vi "Get Level.vi"(6 "Output Channel":T1, 8 "error in (no error)":errorcluster, 11 "Inst.RP100 in":refnum<class "Inst.RP100.lvclass">) -> (0 "error out":errorcluster, 2 "Level (V)":dbl, 3 "Inst.RP100 out":refnum<class "Inst.RP100.lvclass">)   [LabVIEW 2019, in "Inst.RP100.lvclass"]
uses:
  Inst.RP100.lvclass
  C:/Program Files (x86)/National Instruments/LabVIEW 2019/user.lib/LevyLab/Instrument Framework/SMOs/Instrument/Instrument.lvclass
  Typedefs/Output Channel--Enum.ctl
  Typedefs/Commands--Enum.ctl
  Typedefs/getLevel--Cluster.ctl
  <userlib>/LevyLab/Instrument Framework/SMOs/Instrument/Instrument.lvclass/Instrument.ctl
  01165c8c-b2e8-49b8-96e8-536698999359.vi/012e8175-f6b3-4063-807e-eae00dfba7fe.vi
  01165c8c-b2e8-49b8-96e8-536698999359.vi/012e8175-f6b3-4063-807e-eae00dfba7fe.vi/41478f01-57f4-4188-8f0a-c43f95c8f48e.vi
  <userlib>/LevyLab/Instrument Framework/SMOs/Instrument/API/Send and Receive.vi
  01165c8c-b2e8-49b8-96e8-536698999359.vi/012e8175-f6b3-4063-807e-eae00dfba7fe.vi/390a0fe6-66d0-4b1f-8944-62df44ed410c.vi
  <userlib>/LevyLab/Instrument Framework/SMOs/Instrument/Private/Get Client Type.vi
  01165c8c-b2e8-49b8-96e8-536698999359.vi/012e8175-f6b3-4063-807e-eae00dfba7fe.vi/41478f01-57f4-4188-8f0a-c43f95c8f48e.vi/d4522e91-9053-4c0e-9d1f-c7c48f8b6bcc.vi
  01165c8c-b2e8-49b8-96e8-536698999359.vi/012e8175-f6b3-4063-807e-eae00dfba7fe.vi/41478f01-57f4-4188-8f0a-c43f95c8f48e.vi/891fa407-0db4-4b04-91cd-89da5eed44a8.vi
  01165c8c-b2e8-49b8-96e8-536698999359.vi/012e8175-f6b3-4063-807e-eae00dfba7fe.vi/390a0fe6-66d0-4b1f-8944-62df44ed410c.vi/4d54c90f-f017-4dd3-9061-6dca01a9e2e0.vi
  01165c8c-b2e8-49b8-96e8-536698999359.vi/012e8175-f6b3-4063-807e-eae00dfba7fe.vi/390a0fe6-66d0-4b1f-8944-62df44ed410c.vi/c432f00d-fbcb-44ec-80e1-5223097179db.vi
  01165c8c-b2e8-49b8-96e8-536698999359.vi/012e8175-f6b3-4063-807e-eae00dfba7fe.vi/390a0fe6-66d0-4b1f-8944-62df44ed410c.vi/4d54c90f-f017-4dd3-9061-6dca01a9e2e0.vi/4a32ab2b-883d-45ba-8bf7-73b0a157e865.vi
  01165c8c-b2e8-49b8-96e8-536698999359.vi/012e8175-f6b3-4063-807e-eae00dfba7fe.vi/390a0fe6-66d0-4b1f-8944-62df44ed410c.vi/4d54c90f-f017-4dd3-9061-6dca01a9e2e0.vi/9b068e5f-e603-4ccd-b66b-d4bd0b9420a9.vi
  <userlib>/LevyLab/Instrument Framework/SMOs/Instrument/Private/Get RC Connection Status.vi
  <userlib>/LevyLab/Instrument Framework/SMOs/Instrument/API/Enum to String.vi
  <userlib>/LevyLab/Instrument Framework/SMOs/RemoteControl/API/Send and Receive.vi
  <vilib>/Utility/Data Type/Get Type Information.vi
  <vilib>/JDP Science/JSONtext/JSON text to Variant.vi
  <userlib>/LevyLab/Instrument Framework/SMOs/Instrument/API/Instrument.GetPublicEvents.vi
  <vilib>/JDP Science/JSONtext/Variant to JSON Text.vi
  <vilib>/National Instruments/GUID Generator/Guid Generator.vi
  <userlib>/LevyLab/Instrument Framework/SMOs/Instrument/API/Instrument.MessageToProcess.vi
  <userlib>/LevyLab/Instrument Framework/SMOs/Instrument/Private/Instrument.MessageFromProcess.EventStructure.vi
  <vilib>/JDP Science/JSONtext/LVClass Serializer/JSONtext LVClass Serializer.lvclass
  76e71197-b2f6-4e88-bdc7-a729cadb6927.vi
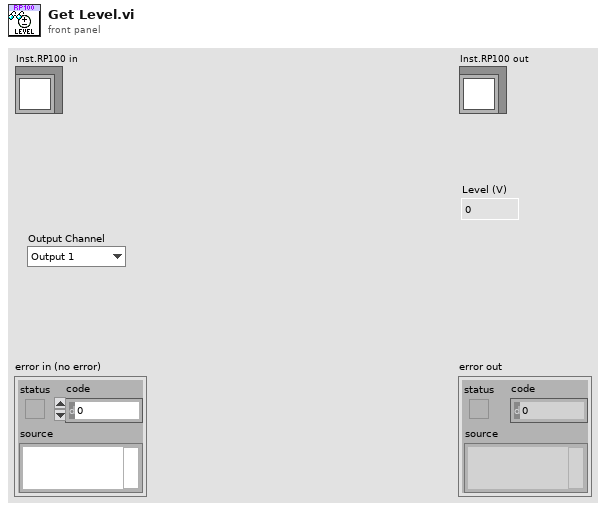
[diagram p1: front panel]
types:
  T1 = typedef "Inst.RP100.lvclass/Output Channel--Enum.ctl" = enum16{"Output 1", "Output 2"}
  T2 = typedef "Inst.RP100.lvclass/getLevel--Cluster.ctl" = cluster{"Channel":T1}
  T3 = typedef "Inst.RP100.lvclass/Commands--Enum.ctl" = enum16{"setState", "setStrain", "getStrain", "setLevel", "getLevel"}
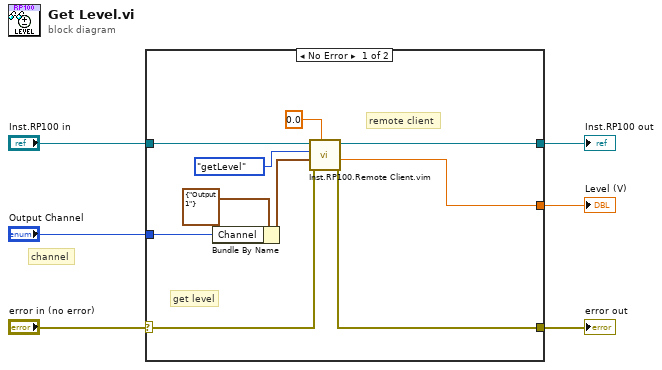
[diagram p0: block diagram]
diagram:
  # "channel"
  n1 = case shown="No Error" "error in (no error)" {
    selector: "error in (no error)" -> [w11 w18]
    tunnel: [w10 w18] -> w5
    tunnel: "Inst.RP100 in" -> [w16 w17]
    tunnel: [w15 w17] -> w3
    tunnel: [w12 _] -> w1
    tunnel: "Output Channel" -> [w8 _]
    frame No Error {
      # "remote client"
      # "get level"
      n2 = Bundle By Name(cluster=T2 {"Channel"=enum."Output 1"} ("getLevel"), "Channel"=w8) -> (w7:T2)
      n3 = call "Inst.RP100.Remote Client.vim"("Data Out type"=0.0, "error in (no error)"=w11, "params"=w7, "Commands"=Commands--Enum."getLevel", "Inst.RP100 in"=w16) -> ("error out"=w10:errorcluster, "Data out"=w12:dbl, "Inst.RP100 out"=w15:refnum<class "Inst.RP100.lvclass">)  [unwired: 4 in]
    }
    frame Error {
    }
  }
  "error out" <- w5
  "Inst.RP100 out" <- w3
  "Level (V)" <- w1
